vi "Get_Shaft_Fundamental.vi"(8 "error in (no error)":errorcluster, 11 "Data Cluster in":T1 {"Shaft"."dmin" format="%#_7g"; "Shaft"."dmax" format="%#_7g"; "Shaft"."Fundamental Dev" format="%#_7g"; "Shaft"."Tolerance Grade (IT) Shaft" format="%#_7g"; "Hole"."Dmin" format="%#_7g"; "Hole"."Tolerance Grade (IT)" format="%#_7g"}) -> (0 "error out":errorcluster, 3 "Data Cluster out":T1 {"Shaft"."dmin" format="%#_7g"; "Shaft"."dmax" format="%#_7g"; "Shaft"."Fundamental Dev" format="%#_7g"; "Shaft"."Tolerance Grade (IT) Shaft" format="%#_7g"; "Hole"."Dmin" format="%#_7g"; "Hole"."Tolerance Grade (IT)" format="%#_7g"})   [LabVIEW 2023]
uses:
  TypeDef/Data_Cluster.ctl
  <vilib>/MGI/Panel Manager/Panel/Panel/Window/Window.lvclass
  TypeDef/Units.ctl
  TypeDef/Method_Info.ctl
  TypeDef/Hole_Data.ctl
  TypeDef/Shaft_Data.ctl
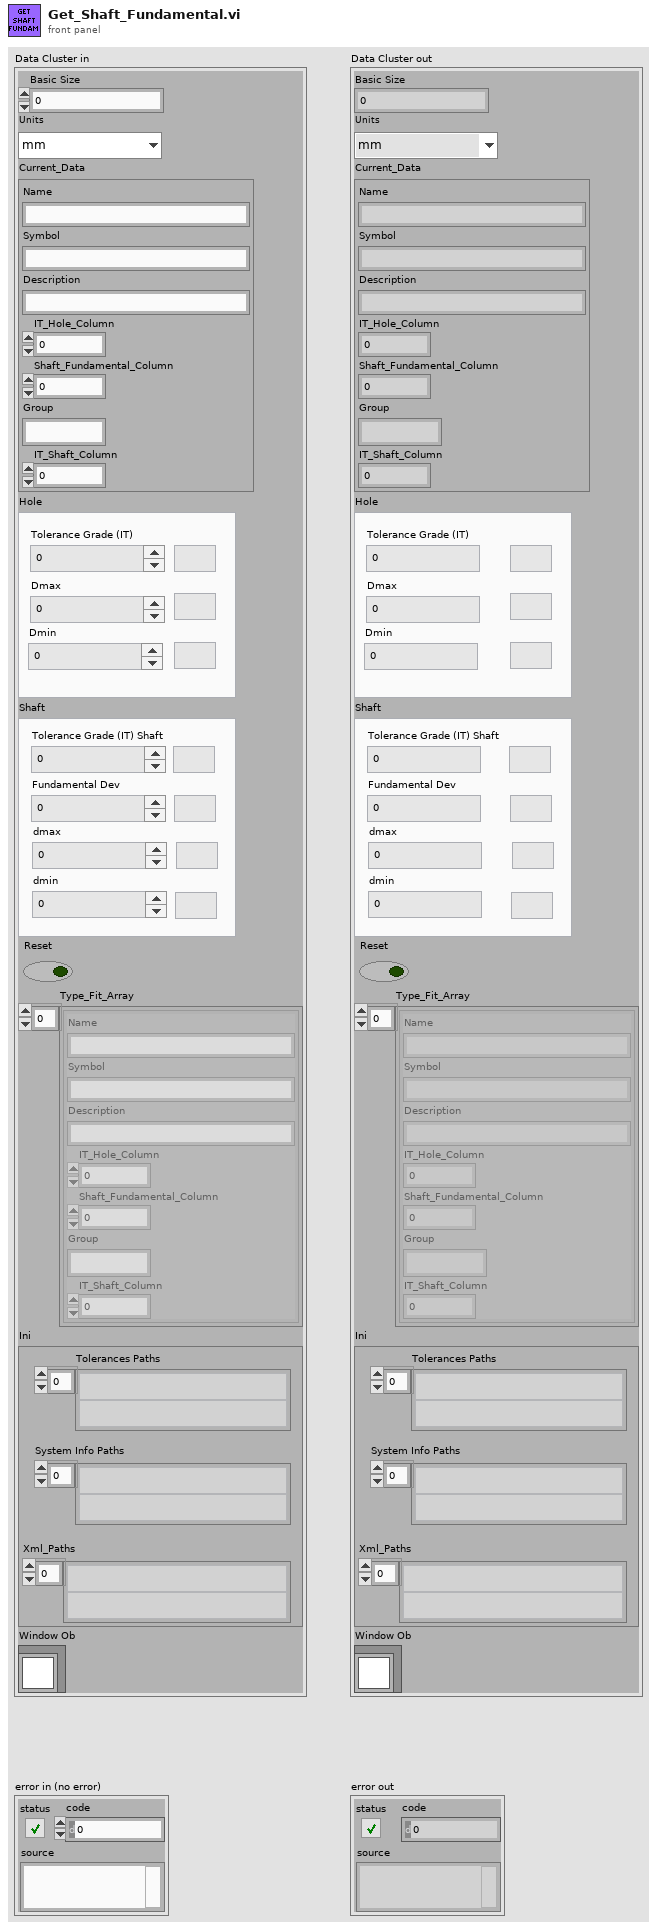
[diagram p1: front panel]
types:
  T1 = typedef "Data_Cluster.ctl" = cluster{"Basic Size ":dbl, "Units":T2, "Current_Data":T3, "Hole":T4, "Shaft":T5, "Reset":bool, "Type_Fit_Array":T3[], "Ini":cluster{"Tolerances Paths":path[], "System Info Paths":path[], "Xml_Paths":path[]}, "Window Ob":refnum<class "Window.lvclass">}
  T2 = typedef "Units.ctl" = enum16{"mm", "in"}
  T3 = typedef "Method_Info.ctl" = cluster{"Name":string, "Symbol":string, "Description":string, "IT_Hole_Column":i32, "Shaft_Fundamental_Column":i32, "Group":string, "IT_Shaft_Column":i32}
  T4 = typedef "Hole_Data.ctl" = cluster{"Tolerance Grade (IT)":dbl, "Dmax":dbl, "Units Hole":cluster{"units_it":string, "units_Dmax\nUnits_Dmax":string, "Units_Dmin":string}, "Dmin":dbl}
  T5 = typedef "Shaft_Data.ctl" = cluster{"Tolerance Grade (IT) Shaft":dbl, "Units Shaft":cluster{"Units_FundamentalDev":string, "Units_dmax":string, "Units_dmin":string, "Units_IT_Shaft":string}, "Fundamental Dev":dbl, "dmax":dbl, "dmin":dbl}
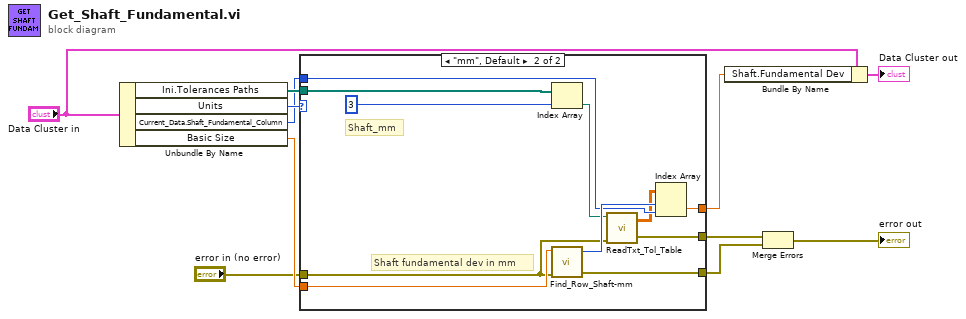
[diagram p0: block diagram]
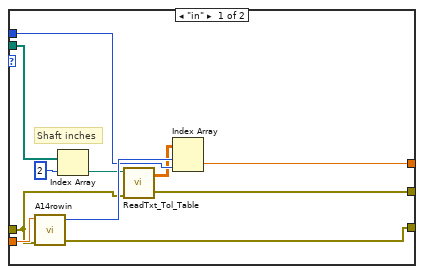
[diagram p2: hidden frame]
diagram:
  n1 = Unbundle By Name("Data Cluster in") -> ("Ini.Tolerances Paths"=w7:path[], "Units"=w2:T2, "Current_Data.Shaft_Fundamental_Column"=w1:i32, "Basic Size"=w8:dbl)
  n2 = case shown="\"mm\", Default" w2 {
    tunnel: w1 -> [w19 w30]
    tunnel: w8 -> [w22 w33]
    tunnel: [w18 w29] -> w9
    tunnel: "error in (no error)" -> [w16 w26]
    tunnel: [w17 w27] -> w4
    tunnel: [w21 w32] -> w6
    tunnel: w7 -> [w13 w24]
    frame "in" {
      # "Shaft inches"
      n3 = call "A14rowin.vi"("Basic Size"=w22, "error in (no error)"=w16) -> ("Row"=w20:i32, "error out"=w21:errorcluster)  [unwired: 5 in]
      n4 = Index Array(array=w13, index=2) -> (element=w14:path)
      n5 = call "ReadTxt_Tol_Table.vi"("error in"=w16, "ITmm path"=w14) -> ("error out"=w17:errorcluster, "array_of_tolerances"=w15:dbl[][])  [unwired: 4 in]
      n6 = Index Array(array=w15, index (row)=w20, index (col)=w19) -> (element=w18:dbl)
    }
    frame "mm", Default {
      # "Shaft_mm"
      # "Shaft fundamental dev in mm"
      n7 = Index Array(array=w24, index=3) -> (element=w25:path)
      n8 = call "Find_Row_Shaft-mm.vi"("Basic Size"=w33, "error in"=w26) -> ("Row"=w31:i32, "error out"=w32:errorcluster)  [unwired: 5 in]
      n9 = call "ReadTxt_Tol_Table.vi"("error in"=w26, "ITmm path"=w25) -> ("error out"=w27:errorcluster, "array_of_tolerances"=w28:dbl[][])  [unwired: 4 in]
      n10 = Index Array(array=w28, index (row)=w31, index (col)=w30) -> (element=w29:dbl)
    }
  }
  n11 = Bundle By Name(cluster="Data Cluster in", "Shaft.Fundamental Dev"=w9) -> (→"Data Cluster out":T1)
  n12 = Merge Errors(w4, w6) -> (→"error out":errorcluster)
